vi "FPGA Draw doodle.vi"   [LabVIEW 2019]
uses:
  <vilib>/rvi/Memory/Memory_Emulation/nirvimemoryFastEmulation.vi
  <vilib>/rvi/Memory/Memory_Emulation/nirvimemoryEmulation.vi
  <vilib>/rvi/Emulation/niFpgaEmulationIsFPGAContextNoSignature.vi
  <vilib>/rvi/DataTransferAndStorage/Container/Common/niFpgaContainerGetUniqueNameForEmu.vi
  <vilib>/rvi/Emulation/niFpgaProcessEmulError.vi
  <vilib>/rvi/Emulation/niFpgaSctlEmulationGetInTimedLoop.vi
  <vilib>/rvi/errors/nirviReportUnexpectedCaseInternalError (U32).vi
  <vilib>/rvi/DataTransferAndStorage/Container/XNode/niFpgaContainer.xnode
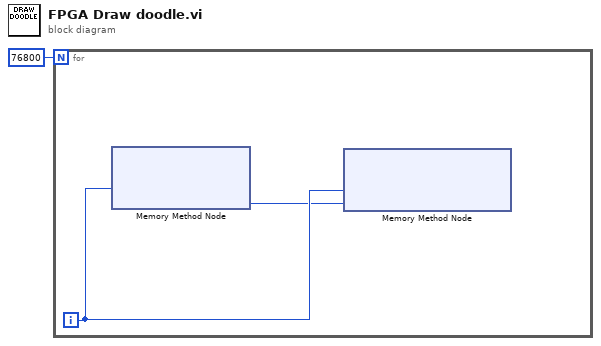
[diagram p0: block diagram]
diagram:
  n1 = for {
    N: 76800 -> [_]
    i -> [w3]
    n2 = xnode ("Memory Method Node")("Address"=w3) -> ("Data"=w2:u16)  [unwired: 1 in, 1 out]
    n3 = xnode ("Memory Method Node")("Address"=w3, "Data"=w2) -> ()  [unwired: 1 in, 1 out]
  }
